vi "Template Dut TxRx Fetch Results.vi"(0 "Dut Handle in":T2, 11 "error in (no error)":errorcluster) -> (4 "Dut Handle out":T2, 8 "Template Results":T1, 15 "error out":errorcluster)   [LabVIEW 2014, in "niDTS Template.lvlib"]
uses:
  niDTS Template.lvlib
  Framework/Dut/Includes/niDTS Dut INC Handle.ctl
  Framework/Dut/Objects/BASE_class/niDTS Dut.lvclass
  Includes/Template Dut INC Results.ctl
  Includes/Template Dut INC Handle.ctl
  Objects/BASE_class/Template Dut.lvclass
  Framework/niDTS Framework.lvlib
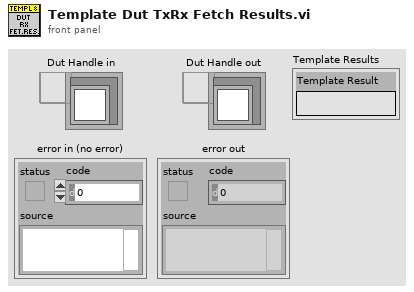
[diagram p1: front panel]
types:
  T1 = typedef "niDTS Template.lvlib/Template Dut INC Results.ctl" = cluster{"Template Result":string}
  T2 = typedef "niDTS Framework.lvlib/niDTS Dut INC Handle.ctl" = refnum<data-value>
  T3 = typedef "niDTS Template.lvlib/Template Dut INC Handle.ctl" = refnum<data-value>
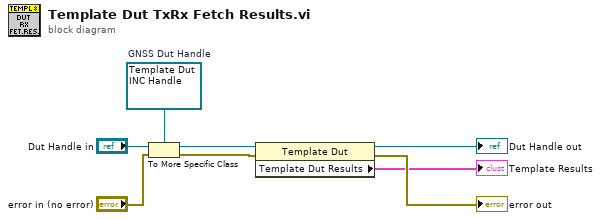
[diagram p0: block diagram]
diagram:
  w6 = T3 refnum  # GNSS Dut Handle
  n1 = To More Specific Class(target class=w6, reference="Dut Handle in", error in="error in (no error)") -> (specific class reference=w5:T3, error out=w4:errorcluster)
  n2 = property class="Template Dut"(reference=w5, error in=w4) -> (reference out=→"Dut Handle out":T3, error out=→"error out":errorcluster, "Template Dut Results"=→"Template Results":T1)
